vi "Tree-ParseRawData.vi"(0 "Raw Data":string[][](array[string])=[["PL-2075-3AH", "Manufacturing                                                                                                                                                                                                                                                  ", "1         ", "Testing this crap", "C:\\Users\\tommyj\\Pictures\\ITS ERP System Pictures\\Admin.jpg                                                                                                                                                                                                     ", "C:\\Users\\tommyj\\Pictures\\ITS ERP System Pictures\\Create Inspection Instruction.png                                                                                                                                                                             ", "C:\\Users\\tommyj\\Pictures\\ITS ERP System Pictures\\Stock Inventory.jpg                                                                                                                                                                                           ", "C:\\Users\\tommyj\\Pictures\\ITS ERP System Pictures\\edit-icon.png                                                                                                                                                                                                 ", "C:\\Users\\tommyj\\Pictures\\ITS ERP System Pictures\\Finished Goods Icon.png                                                                                                                                                                                       ", "C:\\Users\\tommyj\\Pictures\\ITS ERP System Pictures\\Pull From Inventory.jpg                                                                                                                                                                                       ", "C:\\Users\\tommyj\\Pictures\\ITS ERP System Pictures\\manufacturing.png                                                                                                                                                                                             ", "Laster Cutting                                                                                                                                                                                                                                                 "], ["PL-2075-3AH", "", "2", "junk", "", "", "", "", "", "", "", ""], ["PL-2075-3AH", "", "3", "asdfasdfasdf", "", "", "", "", "", "", "", ""], ["PP-4562-320", "", "1", "iiiiiiiiii", "", "", "", "", "", "", "", ""], ["PP-4562-320", "", "2", "oooooooooooo", "", "", "", "", "", "", "", ""], ["PP-4562-320", "", "3", "pppppppppp", "", "", "", "", "", "", "", ""], ["PC-258-4561", "", "1", "kkkkkkkkk", "", "", "", "", "", "", "", ""], ["PC-258-4561", "", "2", "lllllllllllllllh", "", "", "", "", "", "", "", ""], ["PC-258-4561", "", "3", "hhhhhhhhhhhh", "", "", "", "", "", "", "", ""], ["PC-258-4561", "", "4", "mmmmmmmmmmmmm", "", "", "", "", "", "", "", ""]]) -> (1 "Tree Data":T1(array[cluster]))   [LabVIEW 2013, in "ERP-CreateInstructions.lvclass"]
uses:
  ERP-CreateInstructions.lvclass
  <userlib>/_OpenG.lib/array/array.llb/Remove Duplicates from 1D Array (String)__ogtk.vi
  <userlib>/_OpenG.lib/array/array.llb/Search 1D Array (String)__ogtk.vi
  <userlib>/_OpenG.lib/array/array.llb/Index 1D Array Elements (String)__ogtk.vi
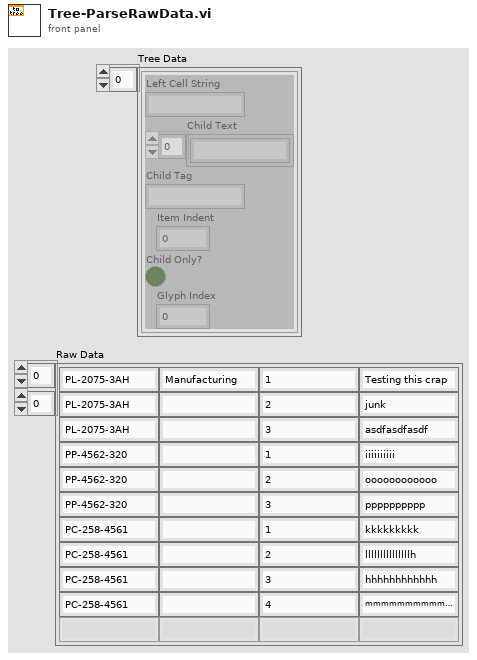
[diagram p1: front panel]
types:
  T1 = cluster{"Left Cell String":string, "Child Text":string[], "Child Tag":string, "Item Indent":i32, "Child Only?":bool, "Glyph Index":i32}[]
  T2 = cluster{"Left Cell String":string, "Child Text":string[], "Child Tag":string, "Item Indent":i32, "Child Only?":bool, "Glyph Index":i32}
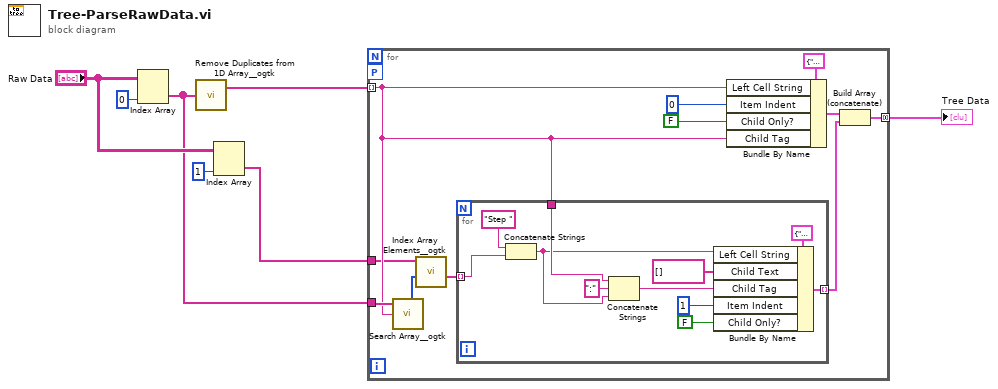
[diagram p0: block diagram]
diagram:
  n1 = Index Array(array="Raw Data", index (col)=0 ("disabled index (col)")) -> (element=w3:string[])  [unwired: 1 in]
  n2 = call-poly <userlib>:"Remove Duplicates from 1D Array__ogtk.vi"("Input Array"=w3) -> ("Output Array"=w1:string[])  [unwired: 1 out]
  n3 = Index Array(array="Raw Data", index (col)=1 ("disabled index (col)")) -> (element=w4:string[])  [unwired: 1 in]
  n4 = for {
    tunnel: [w13] -> w2 mode=concatenating
    tunnel: w1 -> [w11] mode=indexing
    tunnel: w3 -> [w12]
    tunnel: w4 -> [w10]
    workers-P: _ -> [_]
    n5 = call-poly <userlib>:"Search Array__ogtk.vi"("Array"=w12, "Element Data"=w11) -> ("Indices of Elements"=w8:i32[])  [unwired: 7 in]
    n6 = call-poly <userlib>:"Index Array Elements__ogtk.vi"("indices"=w8, "array"=w10) -> ("elements"=w9:string[])  [unwired: 9 in]
    n7 = for {
      tunnel: [w28] -> w14 mode=indexing
      tunnel: w9 -> [w24] mode=indexing
      tunnel: w11 -> [w22]
      n8 = Concatenate Strings("Step " ("string"), w24) -> (w21:string)
      n9 = Concatenate Strings(w22, ":" ("string"), w21) -> (w20:string)
      n10 = Bundle By Name(cluster=T2 {"Left Cell String"="012914", "Child Text"=[], "Child Tag"="", "Item Indent"=0, "Child Only?"=FALSE, "Glyph Index"=0} ("Item"), "Left Cell String"=w21, "Child Text"=string[] [], "Child Tag"=w20, "Item Indent"=1, "Child Only?"=FALSE) -> (w28:T2)
    }
    n11 = Bundle By Name(cluster=T2 {"Left Cell String"="012914", "Child Text"=[], "Child Tag"="", "Item Indent"=0, "Child Only?"=FALSE, "Glyph Index"=0} ("Item"), "Left Cell String"=w11, "Item Indent"=0, "Child Only?"=FALSE, "Child Tag"=w11) -> (w15:T2)
    n12 = Build Array (concatenate)(w15, w14) -> (w13:T1)
  }
  "Tree Data" <- w2
